vi "DFD Arbitrary Group Delay Design.vi"(5 "pole radius constraint":dbl=0.99 min=0.0, 6 "fs [Hz]":dbl=1.0 format="%.2f", 7 "integer offset? (T)":bool=TRUE, 8 "error in (no error)":errorcluster, 10 "band specs":T1[](array[typedef])=[{"subband specs"=[{"freq"=0.0, "group delay"=9.0, "weight"=1.0}, {"freq"=0.2, "group delay"=0.0, "weight"=1.0}]}] {"subband specs"."weight" format="%.2f"}, 11 "order":i32=10) -> (0 "error out":errorcluster, 2 "offset":dbl=-14.0, 3 "filter out":T2={"mSRate_Fs"=1.0, "mSRate_Version"="2.0", "mSRate_Comments"="", "mSRate_OrgCoef"={"type"=enum."Undefined", "gain"=1.0, "coef a (k)"=[], "coef b (v)"=[]}, "mSRate_CurCoef"={"type"=enum."Undefined", "gain"=1.0, "coef a (k)"=[], "coef b (v)"=[]}, "mSRate_Quantized?"=FALSE, "mSRate_QCoef"={"type"=enum."Undefined", "gain"=1.0, "coef a (k)"=[], "coef b (v)"=[]}, "mSRate_QSettings"=[], "mSRate_Order"=0, "mSRate_Scaling"={"mSRate_ScaleByPowerOf2?"=FALSE, "mSRate_ScaleType"=enum."No Norm"}} {"mSRate_QSettings"."source" items=["Coef a/k"=0, "Coef b/v"=7, "Input"=1, "Output"=2, "Multiplicand"=3, "Product"=4, "Sum"=5, "Delay"=6, "Gain"=8]})   [LabVIEW 2017, in "NI_DigFilterLicensed.lvlib"]
doc: "Creates an allpass filter with a group delay that you specify."
uses:
  <vilib>/addons/Digital Filter Design/NI_DigFilterLicensed.lvlib
  <vilib>/addons/Digital Filter Design/_Objects.llb/DFD Filter Obj.ctl
  <vilib>/addons/Digital Filter Design/_Objects.llb/DFD Filter Coef.ctl
  <vilib>/addons/Digital Filter Design/_Objects.llb/DFD Filter Structure Type Selector.ctl
  <vilib>/addons/Digital Filter Design/_Objects.llb/dfd_Internal Quantization Settings.ctl
  <vilib>/addons/Digital Filter Design/_Objects.llb/dfd_Internal Quantization Srcs.ctl
  <vilib>/addons/Digital Filter Design/_Objects.llb/DFD Coef Norm Type.ctl
  <vilib>/addons/Digital Filter Design/_GroupDelay.llb/dfd_Group Delay_Band Spec.ctl
  <vilib>/addons/Digital Filter Design/NI_DigFilter_Design.lvlib
panel:
  # "freq"
  # "group delay"
  # "weight"
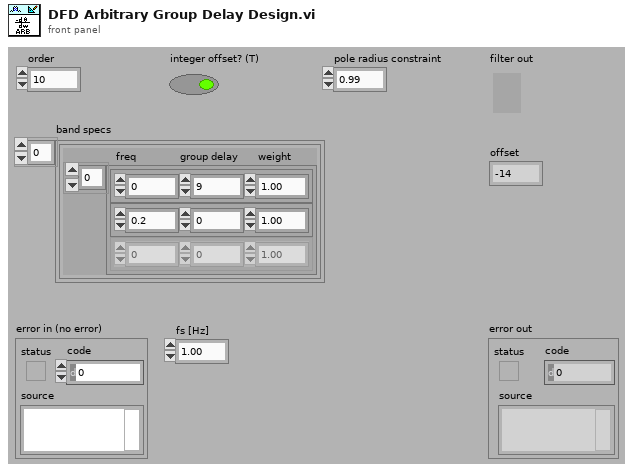
[diagram p1: front panel]
types:
  T1 = typedef "NI_DigFilterLicensed.lvlib/dfd_Group Delay_Band Spec.ctl" = cluster{"subband specs":cluster{"freq":dbl, "group delay":dbl, "weight":dbl}[]}
  T2 = typedef "NI_DigFilterLicensed.lvlib/DFD Filter Obj.ctl" = cluster{"mSRate_Fs":dbl, "mSRate_Version":string, "mSRate_Comments":string, "mSRate_OrgCoef":T3, "mSRate_CurCoef":T3, "mSRate_Quantized?":bool, "mSRate_QCoef":T3, "mSRate_QSettings":T5[], "mSRate_Order":i32, "mSRate_Scaling":cluster{"mSRate_ScaleByPowerOf2?":bool, "mSRate_ScaleType":T7}}
  T3 = typedef "NI_DigFilterLicensed.lvlib/DFD Filter Coef.ctl" = cluster{"type":T4, "gain":dbl, "coef a (k)":dbl[], "coef b (v)":dbl[]}
  T4 = typedef "NI_DigFilterLicensed.lvlib/DFD Filter Structure Type Selector.ctl" = enum16{"Undefined", "FIR Direct Form", "FIR Direct Form Transposed", "FIR Symmetric", "FIR Antisymmetric", "IIR Direct Form I", "IIR Direct Form I Transposed", "IIR Direct Form II", "IIR Direct Form II Transposed", "IIR Cascaded Second Order Sections Form I", "IIR Cascaded Second Order Sections Form I Transposed", "IIR Cascaded Second Order Sections Form II", "IIR Cascaded Second Order Sections Form II Transposed", "Lattice Allpass (basic sections)", "Lattice Allpass (one multiplier sections)", "Lattice Allpass (normalized sections)", "Lattice AR (basic sections)", "Lattice AR (one multiplier sections)", "Lattice AR (normalized sections)", "Lattice MA (minimum phase)", "Lattice MA (maximum phase)", "Lattice ARMA (basic sections)", "Lattice ARMA (one multiplier sections)", "Lattice ARMA (normalized sections)"}
  T5 = typedef "NI_DigFilterLicensed.lvlib/dfd_Internal Quantization Settings.ctl" = cluster{"source":T6, "wl":i16, "iwl":i16, "overflow mode":enum16{"Saturation", "Wrap"}, "rounding mode":enum16{"Nearest", "Truncation"}, "signed?":bool}
  T6 = typedef "NI_DigFilterLicensed.lvlib/dfd_Internal Quantization Srcs.ctl" = u16
  T7 = typedef "NI_DigFilterLicensed.lvlib/DFD Coef Norm Type.ctl" = enum16{"No Norm", "Time Domain 1-Norm", "Time Domain 2-Norm", "Time Domain Inf-Norm"}
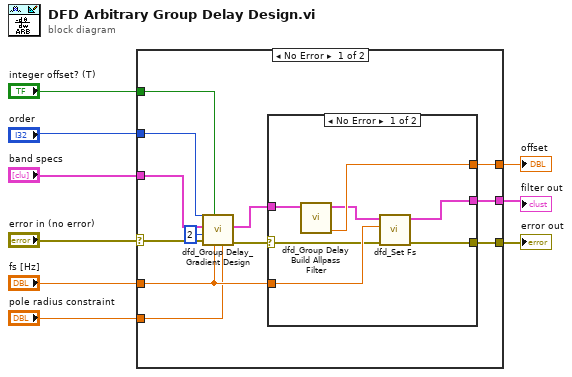
[diagram p0: block diagram]
diagram:
  n1 = case shown="No Error" "error in (no error)" {
    selector: "error in (no error)" -> [w10 w30]
    tunnel: "order" -> [w21 _]
    tunnel: "fs [Hz]" -> [w20 _]
    tunnel: "band specs" -> [w19 _]
    tunnel: "pole radius constraint" -> [w18 _]
    tunnel: [w17 _] -> w5
    tunnel: "integer offset? (T)" -> [w16 _]
    tunnel: [w15 _] -> w3
    tunnel: [w11 w30] -> w2
    frame No Error {
      n2 = call <vilib>:"dfd_Group Delay_Gradient Design.vi"("radius"=w18, "fs (Hz)"=w20, "integer tau?"=w16, "error in (no error)"=w10, "P"=2 ("p"), "band specification"=w19, "order"=w21) -> ("error out"=w12:errorcluster, "Coefficients"=w14:cluster{"r":dbl[], "theta":dbl[], "offset":dbl})  [unwired: 1 in, 2 out]
      n3 = case shown="No Error" w12 {
        selector: w12 -> [w23 w29]
        tunnel: [w22 w29] -> w11
        tunnel: w20 -> [w28 _]
        tunnel: [w27 _] -> w17
        tunnel: [w26 _] -> w15
        tunnel: w14 -> [w25 _]
        frame No Error {
          n4 = call <vilib>:"dfd_Group Delay Build Allpass Filter.vi"("Coefficients"=w25) -> ("offset"=w26:dbl, "filter out"=w24:T2)  [unwired: 9 out]
          n5 = call <vilib>:"dfd_Set Fs.vi"("error in (no error)"=w23, "fs [Hz]"=w28, "filter in"=w24) -> ("error out"=w22:errorcluster, "filter out"=w27:T2)  [unwired: 7 out]
        }
        frame Error {
        }
      }
    }
    frame Error {
    }
  }
  "filter out" <- w5
  "error out" <- w2
  "offset" <- w3
